vi "Autonomous.vi"(11 "Call Context":T4) -> (5 "SubState 0":T2=enum."driver control", 7 "Loop 0 Data":T1, 10 "SubState 1":T3)   [LabVIEW 2013]
uses:
  typedefs/subStates.ctl
  <vilib>/Rock Robotics/WPI/DriverStation/WPI_DriverStationDerivedRobotMode.ctl
  typedefs/singleUseSubstate.ctl
  typedefs/Loop Datatypes/Loop 0 Datatype.ctl
  typedefs/fg_typedef.ctl
  typedefs/vision enable.ctl
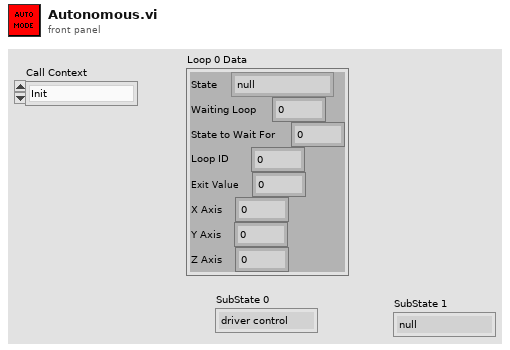
[diagram p1: front panel]
types:
  T1 = typedef "Loop 0 Datatype.ctl" = cluster{"State":T2, "Waiting Loop":i32, "State to Wait For":i32, "Loop ID":i32, "Exit Value":i32, "X Axis":dbl, "Y Axis":dbl, "Z Axis":dbl}
  T2 = typedef "subStates.ctl" = enum16{"null", "wait", "driver control", "auto", "manual override", "hold position", "rotate", "pickup", "pass", "load", "goto shoot", "shoot", "end"}
  T3 = typedef "singleUseSubstate.ctl" = enum16{"null", "wait", "shift high", "shift low"}
  T4 = typedef "WPI_DriverStationDerivedRobotMode.ctl" = enum16{"Init", "Execute", "Stop"}
  T5 = typedef "vision enable.ctl" = enum16{"Enable", "Disable", "Stop"}
  T6 = typedef "fg_typedef.ctl" = enum16{"Get", "Set"}
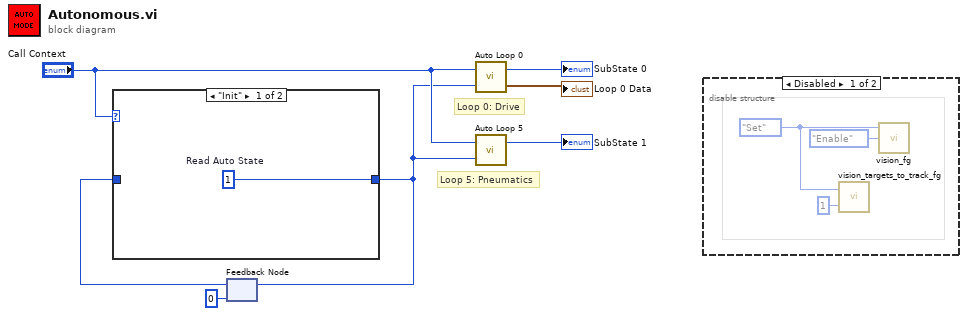
[diagram p0: block diagram]
diagram:
  # "Loop 5: Pneumatics"
  # "Loop 0: Drive"
  n1 = feedback #1(u8 0 ("Read Auto State")) -> (w1:u8)
  n2 = case shown="\"Init\"" "Call Context" {
    tunnel: [w8 w9] -> w3
    tunnel: w1 -> [_ w9]
    frame "Init" {
      w8 = u8 1  # Read Auto State
    }
    frame "Execute", Default {
    }
  }
  n3 = feedback-in #1(w3) -> ()
  n4 = call "Auto Loop 0.vi"("Auto State"=w3, "Call Context"="Call Context") -> ("Loop 0 Data"=→"Loop 0 Data":T1, "SubState 0"=→"SubState 0":T2)
  n5 = call "Auto Loop 5.vi"("Auto State"=w3, "Call Context"="Call Context") -> ("SubState 5"=→"SubState 1":T3)  [unwired: 1 in]
  n6 = disable-structure shown="Disabled" {
    frame Disabled {
      w12 = fg_typedef."Set" ("Menu")
      n7 = call "vision_targets_to_track_fg.vi"("Input"=1, "Menu (Get)"=w12) -> ()  [unwired: 1 out]
      n8 = call "vision_fg.vi"("Action"=vision_enable."Enable", "Menu"=w12) -> ()  [unwired: 1 in, 2 out]
    }
    frame Enabled {
    }
  }
